vi "VCSV-Code-Program.vi"() -> ()   [LabVIEW 2018]
uses:
  <vilib>/sound2/lvsound2.llb/Sound Data Format.ctl
  <vilib>/sound2/lvsound2.llb/Sampling Mode.ctl
  <vilib>/userdefined/High Color/IMAQdx.ctl
  <vilib>/Analysis/3filter.llb/Filter Passband Type.ctl
  <vilib>/Analysis/2dsp.llb/Real FFT.vi
  <vilib>/Analysis/2dsp.llb/Inverse Real FFT.vi
  <vilib>/sound2/lvsound2.llb/Sound Input Read (DBL).vi
  <vilib>/Analysis/3filter.llb/Butterworth Filter (DBL).vi
  <vilib>/imath/engines/lvmath2/RunTimeEngine/BuiltInFunctions/length/NIMS_length(GV).vi
  <instcachedir>/0/NIMS_length(GV)_08A3D13377FD4E4B96F5795FBF3698FA.lvgen/NIMS_length(GV)_08A3D13377FD4E4B96F5795FBF3698FA_000.vi
  <vilib>/imath/engines/lvmath2/RunTimeEngine/CommandStatement/MC_CommandStatement_break.vi
  <vilib>/imath/engines/lvmath2/RunTimeEngine/IndexRead/NIMS V(S).vi
  <instcachedir>/0/NIMS V(S)_0488751826AF41519A22953C041130DC.lvgen/NIMS V(S)_0488751826AF41519A22953C041130DC_000.vi
  <vilib>/imathl/engines/lvmath/Functions/Error Handling/Create Error.vi
  <vilib>/imath/engines/lvmath2/RunTimeEngine/CommandStatement/NIMS_CommandStatement_MaskErr.vi
  <vilib>/imath/engines/lvmath2/RunTimeEngine/NodeEndStatement/NIMS_NodeEndStatement_Output.vi
  <instcachedir>/0/NIMS_NodeEndStatement_Output_53EC0D466D134D7ABD903AC30B43404B.lvgen/NIMS_NodeEndStatement_Output_53EC0D466D134D7ABD903AC30B43404B_010.vi
  <instcachedir>/0/NIMS_NodeEndStatement_Output_53EC0D466D134D7ABD903AC30B43404B.lvgen/NIMS_NodeEndStatement_Output_53EC0D466D134D7ABD903AC30B43404B_009.vi
  <vilib>/imath/engines/lvmath2/RunTimeEngine/ErrorHandling/NIMS_Finalize Error.vi
  <vilib>/Analysis/2dsp.llb/Zero Padder (DBL).vi
  <vilib>/imath/engines/lvmath2/RunTimeEngine/Managers/WorkSpace/UID Generator.vi
  <vilib>/imath/engines/lvmath2/RunTimeEngine/RunTimeType/NIMS_RunTimeType_From StrictType (excl LVString).vi
  <instcachedir>/0/NIMS_RunTimeType_From StrictType (excl LVString)_E7E34A65C99947108168652BAD14964D.lvgen/NIMS_RunTimeType_From StrictType (excl LVString)_E7E34A65C99947108168652BAD14964D_000.vi
  <vilib>/imath/engines/lvmath2/RunTimeEngine/LocalVariableDefStatement/MC_LocalVariableDefStatement_Display.vi
  <vilib>/imath/engines/lvmath2/RunTimeEngine/Managers/SymbolTable/Clear UID.vi
  <vilib>/Analysis/NI_AALBase.lvlib
  <vilib>/Analysis/NI_AALPro.lvlib
  <vilib>/imath/engines/lvmath2/RunTimeEngine/Managers/SymbolTable/NIMS_WorkSpace.lvlib
  <vilib>/vision/driver/NI_Vision_Acquisition_Software.lvlib
panel:
  in  "temp":dbl=25.0
  in  "stop":bool
  out "X":dbl
  out "Y":dbl
  out "Z":dbl
  out "theta":dbl
  out "phi":dbl
  out "c 2":i32
  in  "Hide/Show (Show)":bool=TRUE
  in  "Bring To Front? (N)":bool
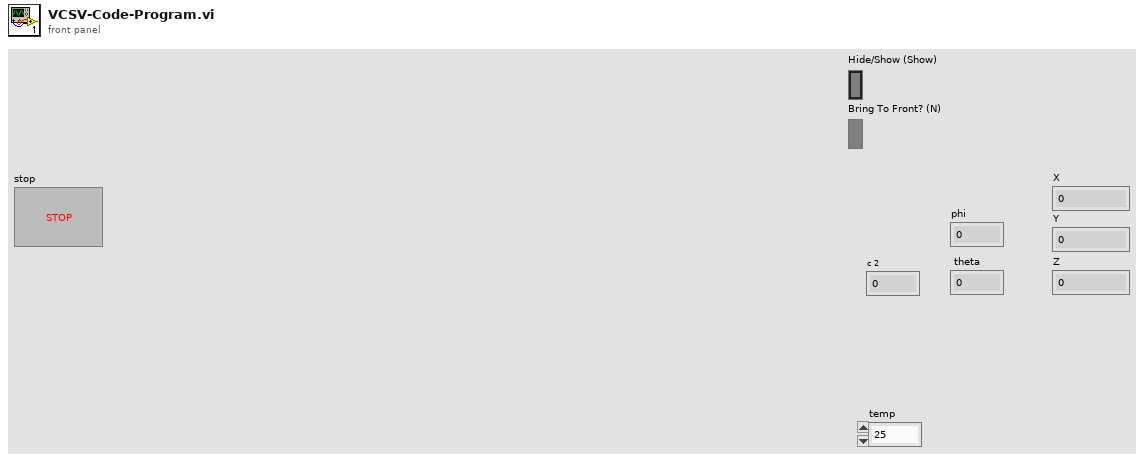
[diagram p1: front panel]
types:
  T1 = typedef "IMAQdx.ctl" = refnum<k21>
  T2 = typedef "Sampling Mode.ctl" = i32
  T3 = typedef "Sound Data Format.ctl" = cluster{"sample rate (S/s)":dbl, "number of channels":i32, "bits per sample":i32}
  T4 = typedef "Sound Input Task ID.ctl" = u32
  T5 = typedef "NI_AALBase.lvlib/Filter Passband Type.ctl" = enum32{"Lowpass", "Highpass", "Bandpass", "Bandstop"}
  T6 = typedef "IMAQ Image.ctl" = refnum<image>
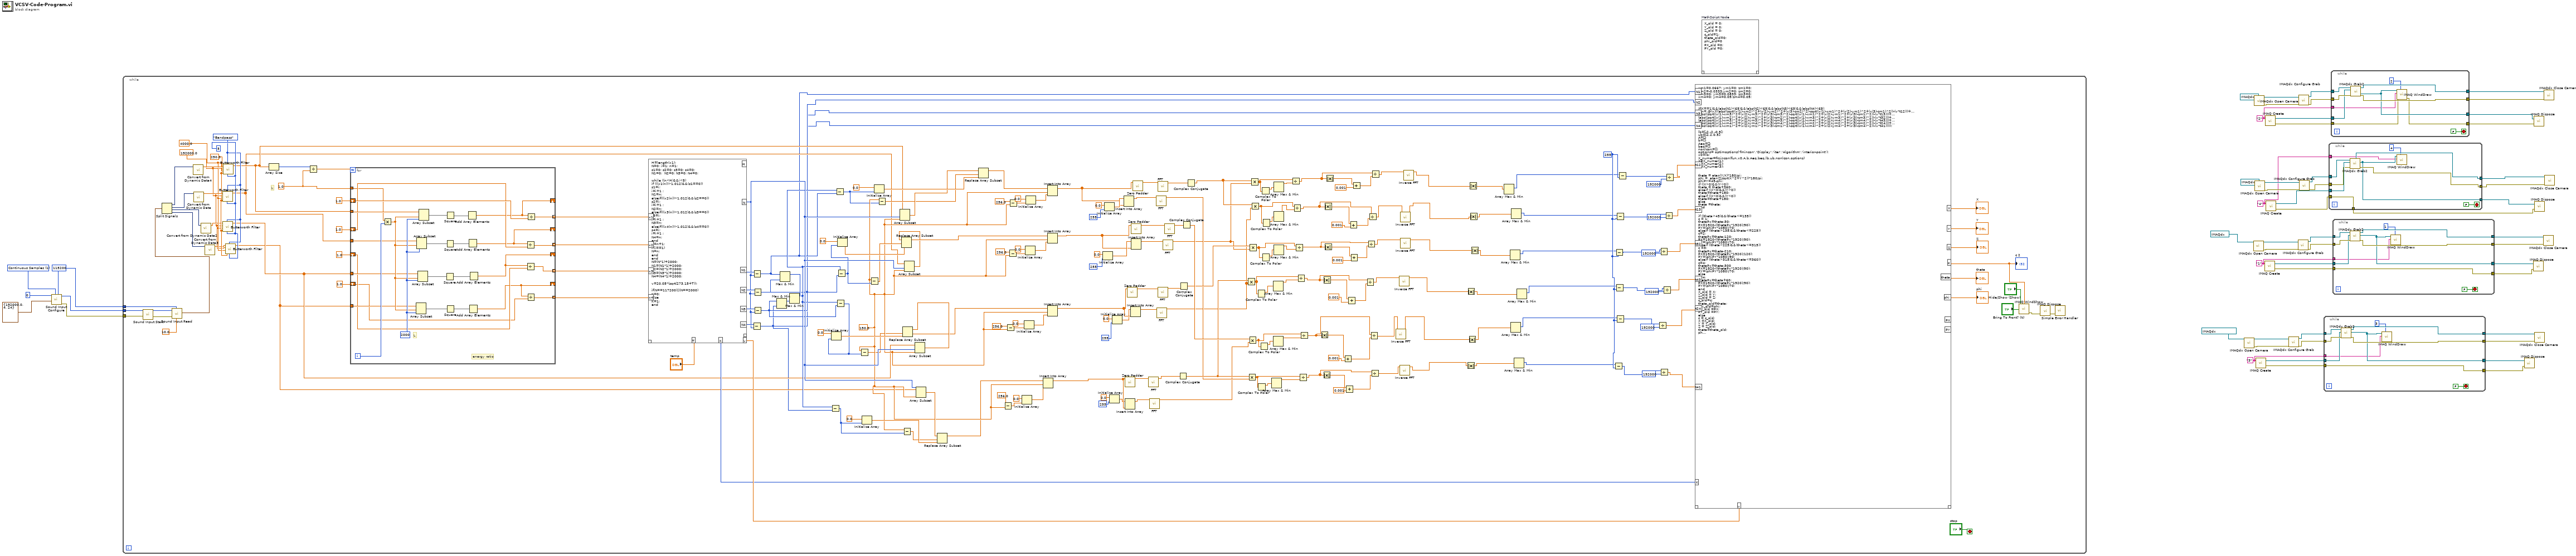
[diagram p0: block diagram]
diagram:
  w1 = "3" ("Image Name")
  w15 = "2" ("Image Name")
  w14 = "4" ("Image Name")
  w13 = "1" ("Image Name")
  w53 = T2 1 items=["Finite Samples", "Continuous Samples"] ("sample mode")
  w51 = 115200 ("number of samples/ch")
  n1 = call <vilib>:"Sound Input Configure.vi"("number of samples/ch"=w51, "sample mode"=w53, "sound format"=T3 {"sample rate (S/s)"=192000.0, "number of channels"=4, "bits per sample"=24}, "device ID"=u32 0) -> ("error out"=w50:errorcluster, "task ID"=w49:T4)  [unwired: 6 in]
  n2 = while {
    tunnel: w51 -> [w272]
    tunnel: w50 -> [w271]
    tunnel: w49 -> [w270]
    stop <- "stop" stop-if-true
    w65 = 1.0 ("x")
    w119 = 150.0
    w150 = 4000.0 ("high cutoff freq: fh")
    w151 = 250.0 ("low cutoff freq: fl")
    w152 = 5 ("order")
    w147 = 192000.0 ("sampling freq: fs")
    w146 = Filter_Passband_Type."Bandpass" ("filter type")
    w164 = 255
    # "k"
    n3 = call <vilib>:"Sound Input Start.vi"("error in (no error)"=w271, "task ID"=w270) -> ("error out"=w275:errorcluster, "task ID out"=w274:T4)  [unwired: 8 in]
    n4 = call-poly <vilib>:"Sound Input Read.vi"("timeout (sec)"=10.0, "number of samples/ch"=w272, "error in (no error)"=w275, "task ID"=w274) -> ("data"=w157:waveform(dbl)[])  [unwired: 5 in, 2 out]
    n5 = Split Signals(w157) -> (w277:dynamicdata, w156:dynamicdata, w155:dynamicdata, w158:dynamicdata)  [unwired: 4 in]
    n6 = call "Convert from Dynamic Data4"("Dynamic Data Type"=w277) -> ("Array"=w154:dbl[])  [unwired: 3 in]
    n7 = call "Convert from Dynamic Data"("Dynamic Data Type"=w156) -> ("Array"=w153:dbl[])  [unwired: 3 in]
    n8 = call "Convert from Dynamic Data2"("Dynamic Data Type"=w155) -> ("Array"=w149:dbl[])  [unwired: 3 in]
    n9 = call "Convert from Dynamic Data3"("Dynamic Data Type"=w158) -> ("Array"=w148:dbl[])  [unwired: 3 in]
    n10 = call-poly <vilib>:"Butterworth Filter.vi"("order"=w152, "filter type"=w146, "low cutoff freq: fl"=w151, "high cutoff freq: fh"=w150, "sampling freq: fs"=w147, "X"=w153) -> ("Filtered X"=w99:dbl[])  [unwired: 2 in, 1 out]
    n11 = call-poly <vilib>:"Butterworth Filter.vi"("order"=w152, "filter type"=w146, "low cutoff freq: fl"=w151, "high cutoff freq: fh"=w150, "sampling freq: fs"=w147, "X"=w149) -> ("Filtered X"=w98:dbl[])  [unwired: 2 in, 1 out]
    n12 = call-poly <vilib>:"Butterworth Filter.vi"("order"=w152, "filter type"=w146, "low cutoff freq: fl"=w151, "high cutoff freq: fh"=w150, "sampling freq: fs"=w147, "X"=w154) -> ("Filtered X"=w100:dbl[])  [unwired: 2 in, 1 out]
    n13 = call-poly <vilib>:"Butterworth Filter.vi"("order"=w152, "filter type"=w146, "low cutoff freq: fl"=w151, "high cutoff freq: fh"=w150, "sampling freq: fs"=w147, "X"=w148) -> ("Filtered X"=w97:dbl[])  [unwired: 2 in, 1 out]
    n14 = Array Size(array=w100) -> (size(s)=w66:i32)
    n15 = Divide(x=w66, y=w65) -> (x/y=w64:dbl)
    n16 = for {
      N: w64 -> [_]
      tunnel: w100 -> [w305]
      shift-right: [w285] -> _
      shift-left: 1.0 -> [w304]
      tunnel: [w303] -> w104 mode=indexing
      tunnel: w99 -> [w296]
      tunnel: w98 -> [w297]
      tunnel: w97 -> [w298]
      shift-right: [w283] -> _
      shift-left: 1.0 -> [w292]
      tunnel: [w291] -> w103 mode=indexing
      shift-right: [w281] -> _
      shift-left: 1.0 -> [w290]
      tunnel: [w289] -> w102 mode=indexing
      shift-right: [w279] -> _
      shift-left: 1.0 -> [w287]
      tunnel: [w288] -> w101 mode=indexing
      tunnel: w65 -> [w278]
      i -> [w301]
      w300 = 2000 ("length")
      # "energy ratio"
      # "L"
      n17 = Multiply(x=w278, y=w301) -> (x*y=w299:dbl)
      n18 = Array Subset "Array Subset"(array=w298, index=w299, length=w300) -> (w293:dbl[])
      n19 = Array Subset "Array Subset"(array=w296, index=w299, length=w300) -> (w295:dbl[])
      n20 = Array Subset "Array Subset"(array=w297, index=w299, length=w300) -> (w294:dbl[])
      n21 = Array Subset "Array Subset"(array=w305, index=w299, length=w300) -> (w302:dbl[])
      n22 = Square(x=w294) -> (x^2=w282:dbl[])
      n23 = Square(x=w295) -> (x^2=w284:dbl[])
      n24 = Square(x=w302) -> (x^2=w286:dbl[])
      n25 = Square(x=w293) -> (x^2=w280:dbl[])
      n26 = Add Array Elements(numeric array=w286) -> (sum=w285:dbl)
      n27 = Add Array Elements(numeric array=w284) -> (sum=w283:dbl)
      n28 = Add Array Elements(numeric array=w280) -> (sum=w279:dbl)
      n29 = Add Array Elements(numeric array=w282) -> (sum=w281:dbl)
      n30 = Divide(x=w283, y=w292) -> (x/y=w291:dbl)
      n31 = Divide(x=w281, y=w290) -> (x/y=w289:dbl)
      n32 = Divide(x=w279, y=w287) -> (x/y=w288:dbl)
      n33 = Divide(x=w285, y=w304) -> (x/y=w303:dbl)
    }
    n34 = mathscript code="H=length(x1);\nN=0; i=1; n=1;\ns1=0; s2=0; s3=0; s4=0;\nN1=0;  N2=0; N3=0; N4=0;\n\nwhile ((n<H)&&i<5)\nif (((x1(n))>1.012)&&(s1==0))\ns1=i;\ni=i+1 ;\nN1=n;\nelseif(((x2(n))>1.012)&&(s2==0))\ns2=i;\ni=i+1 ;\nN2=n;\nelseif(((x3(n))>1.012)&&(s3==0))\ns3=i;\ni=i+1 ;\nN3=n;\nelseif(((x4(n))>1.012)&&(s4==0))\ns4=i;\ni=i+1 ;\nN4=n;\nend\nn=n+1;\nif(i==1)\nN=n;\nend\nend\nN=(N*1)+2000;\nN1=(N1*1)+2000;\nN2=(N2*1)+2000;\nN3=(N3*1)+2000;\nN4=(N4*1)+2000;\n\nv=20.05*(sqrt(273.15+T));\n\nif(N==117200)||(N==2000)\nK=0;\nelse\nK=1;\nend"("x1"=w104, "x2"=w103, "x3"=w102, "x4"=w101, "T"="temp") -> ("N"=w128:i32, "v"=w145:cdb, "N1"=w132:i32, "N2"=w131:i32, "N3"=w130:i32, "N4"=w129:i32, "K"=w111:i32)  [unwired: 1 in, 2 out]
    n35 = Subtract(x=w129, y=w128) -> (x-y=w67:i32)
    n36 = Subtract(x=w132, y=w128) -> (x-y=w70:i32)
    n37 = Subtract(x=w131, y=w128) -> (x-y=w69:i32)
    n38 = Subtract(x=w130, y=w128) -> (x-y=w68:i32)
    n39 = Max & Min(x=w68, y=w67) -> (max(x,y)=w127:i32)  [unwired: 1 out]
    n40 = Max & Min(x=w70, y=w69) -> (max(x,y)=w126:i32)  [unwired: 1 out]
    n41 = Max & Min(x=w126, y=w127) -> (max(x,y)=w125:i32)  [unwired: 1 out]
    n42 = Subtract(x=w125, y=w67) -> (x-y=w124:i32)
    n43 = Subtract(x=w125, y=w70) -> (x-y=w118:i32)
    n44 = Subtract(x=w125, y=w68) -> (x-y=w122:i32)
    n45 = Initialize Array "Initialize Array"(0.0 ("element"), w122) -> (w137:dbl[])
    n46 = Subtract(x=w125, y=w69) -> (x-y=w121:i32)
    n47 = Initialize Array "Initialize Array"(0.0 ("element"), w121) -> (w139:dbl[])
    n48 = Subtract(x=w119, y=w122) -> (x-y=w116:dbl)
    n49 = Initialize Array "Initialize Array"(0.0 ("element"), w124) -> (w133:dbl[])
    n50 = Subtract(x=w119, y=w121) -> (x-y=w120:dbl)
    n51 = Initialize Array "Initialize Array"(0.0 ("element"), w118) -> (w142:dbl[])
    n52 = Subtract(x=w119, y=w118) -> (x-y=w117:dbl)
    n53 = Array Subset "Array Subset"(array=w100, index=w128, length=w119) -> (w141:dbl[])
    n54 = Subtract(x=w119, y=w124) -> (x-y=w123:dbl)
    n55 = Array Subset "Array Subset"(array=w99, index=w128, length=w119) -> (w105:dbl[])
    n56 = Replace Array Subset(array=w105, new element=w139, index=w120) -> (w113:dbl[])
    n57 = Array Subset "Array Subset"(array=w98, index=w128, length=w119) -> (w134:dbl[])
    n58 = Replace Array Subset(array=w134, new element=w137, index=w116) -> (w114:dbl[])
    n59 = Array Subset "Array Subset"(array=w97, index=w128, length=w119) -> (w135:dbl[])
    n60 = Replace Array Subset "Replace Array Subset"(array=w135, new element=w133, index=w123) -> (w115:dbl[])
    n61 = Replace Array Subset "Replace Array Subset"(array=w141, new element=w142, index=w117) -> (w112:dbl[])
    n62 = Subtract(x=256.0, y=w119) -> (x-y=w267:dbl)
    n63 = Subtract(x=256.0, y=w119) -> (x-y=w268:dbl)
    n64 = Subtract(x=256.0, y=w119) -> (x-y=w266:dbl)
    n65 = Subtract(x=256.0, y=w119) -> (x-y=w269:dbl)
    n66 = Initialize Array(0.0 ("element"), w267) -> (w254:dbl[])
    n67 = Initialize Array(0.0 ("element"), w268) -> (w257:dbl[])
    n68 = Initialize Array(0.0 ("element"), w266) -> (w256:dbl[])
    n69 = Initialize Array(0.0 ("element"), w269) -> (w255:dbl[])
    n70 = Insert Into Array "Insert Into Array"(array=w115, index=w119, new element=w254) -> (w234:dbl[])
    n71 = Insert Into Array(array=w113, index=w119, new element=w256) -> (w238:dbl[])
    n72 = Insert Into Array(array=w112, index=w119, new element=w255) -> (w252:dbl[])
    n73 = Insert Into Array(array=w114, index=w119, new element=w257) -> (w236:dbl[])
    n74 = Initialize Array(0.0 ("element"), 255 ("dimension size")) -> (w239:dbl[])
    n75 = Initialize Array(0.0 ("element"), 255 ("dimension size")) -> (w253:dbl[])
    n76 = Initialize Array(0.0 ("element"), 255 ("dimension size")) -> (w233:dbl[])
    n77 = Initialize Array(0.0 ("element"), 255 ("dimension size")) -> (w235:dbl[])
    n78 = Insert Into Array(array=w253, new element=w252) -> (w242:dbl[])  [unwired: 1 in]
    n79 = call-poly <vilib>:"Zero Padder.vi"("Input Array"=w234) -> ("Zero Padded Array"=w230:dbl[])  [unwired: 10 in]
    n80 = Insert Into Array(array=w233, new element=w234) -> (w232:dbl[])  [unwired: 1 in]
    n81 = call-poly <vilib>:"Zero Padder.vi"("Input Array"=w236) -> ("Zero Padded Array"=w237:dbl[])  [unwired: 10 in]
    n82 = Insert Into Array(array=w235, new element=w236) -> (w231:dbl[])  [unwired: 1 in]
    n83 = call-poly <vilib>:"Zero Padder.vi"("Input Array"=w238) -> ("Zero Padded Array"=w241:dbl[])  [unwired: 10 in]
    n84 = Insert Into Array(array=w239, new element=w238) -> (w240:dbl[])  [unwired: 1 in]
    n85 = call-poly <vilib>:"Zero Padder.vi"("Input Array"=w252) -> ("Zero Padded Array"=w243:dbl[])  [unwired: 10 in]
    n86 = call-poly <vilib>:"FFT.vi"("X"=w230) -> ("FFT {X}"=w228:cdb[])  [unwired: 9 in, 1 out]
    n87 = call-poly <vilib>:"FFT.vi"("X"=w232) -> ("FFT {X}"=w213:cdb[])  [unwired: 9 in, 1 out]
    n88 = call-poly <vilib>:"FFT.vi"("X"=w242) -> ("FFT {X}"=w215:cdb[])  [unwired: 9 in, 1 out]
    n89 = call-poly <vilib>:"FFT.vi"("X"=w231) -> ("FFT {X}"=w214:cdb[])  [unwired: 9 in, 1 out]
    n90 = call-poly <vilib>:"FFT.vi"("X"=w243) -> ("FFT {X}"=w229:cdb[])  [unwired: 9 in, 1 out]
    n91 = call-poly <vilib>:"FFT.vi"("X"=w237) -> ("FFT {X}"=w227:cdb[])  [unwired: 9 in, 1 out]
    n92 = call-poly <vilib>:"FFT.vi"("X"=w240) -> ("FFT {X}"=w110:cdb[])  [unwired: 9 in, 1 out]
    n93 = call-poly <vilib>:"FFT.vi"("X"=w241) -> ("FFT {X}"=w226:cdb[])  [unwired: 9 in, 1 out]
    n94 = Complex Conjugate(1:w228) -> (0:w217:cdb[])
    n95 = Complex Conjugate(1:w227) -> (0:w218:cdb[])
    n96 = Complex Conjugate(1:w226) -> (0:w219:cdb[])
    n97 = Complex Conjugate(1:w229) -> (0:w216:cdb[])
    n98 = Multiply(x=w217, y=w214) -> (x*y=w207:cdb[])
    n99 = Multiply(x=w217, y=w215) -> (x*y=w212:cdb[])
    n100 = Multiply(x=w219, y=w213) -> (x*y=w209:cdb[])
    n101 = Multiply(x=w218, y=w110) -> (x*y=w205:cdb[])
    n102 = Multiply(x=w216, y=w110) -> (x*y=w201:cdb[])
    n103 = Multiply(x=w216, y=w214) -> (x*y=w203:cdb[])
    n104 = Complex To Polar(r * e^(i*theta)=w207) -> (r=w223:dbl[])  [unwired: 1 out]
    n105 = Complex To Polar(r * e^(i*theta)=w212) -> (r=w225:dbl[])  [unwired: 1 out]
    n106 = Complex To Polar(r * e^(i*theta)=w209) -> (r=w224:dbl[])  [unwired: 1 out]
    n107 = Complex To Polar(r * e^(i*theta)=w201) -> (r=w220:dbl[])  [unwired: 1 out]
    n108 = Complex To Polar(r * e^(i*theta)=w205) -> (r=w222:dbl[])  [unwired: 1 out]
    n109 = Complex To Polar(r * e^(i*theta)=w203) -> (r=w221:dbl[])  [unwired: 1 out]
    n110 = Array Max & Min(array=w225) -> (max value=w211:dbl)  [unwired: 3 out]
    n111 = Array Max & Min(array=w223) -> (max value=w208:dbl)  [unwired: 3 out]
    n112 = Array Max & Min(array=w224) -> (max value=w210:dbl)  [unwired: 3 out]
    n113 = Array Max & Min(array=w220) -> (max value=w202:dbl)  [unwired: 3 out]
    n114 = Array Max & Min(array=w221) -> (max value=w204:dbl)  [unwired: 3 out]
    n115 = Array Max & Min(array=w222) -> (max value=w206:dbl)  [unwired: 3 out]
    n116 = Divide(x=w201, y=w202) -> (x/y=w199:cdb[])
    n117 = Divide(x=w203, y=w204) -> (x/y=w194:cdb[])
    n118 = Divide(x=w205, y=w206) -> (x/y=w195:cdb[])
    n119 = Divide(x=w207, y=w208) -> (x/y=w196:cdb[])
    n120 = Divide(x=w212, y=w211) -> (x/y=w198:cdb[])
    n121 = Divide(x=w209, y=w210) -> (x/y=w197:cdb[])
    n122 = Absolute Value(x=w197) -> (abs(x)=w187:dbl[])
    n123 = Absolute Value(x=w198) -> (abs(x)=w185:dbl[])
    n124 = Absolute Value(x=w196) -> (abs(x)=w189:dbl[])
    n125 = Absolute Value(x=w194) -> (abs(x)=w193:dbl[])
    n126 = Absolute Value(x=w195) -> (abs(x)=w191:dbl[])
    n127 = Absolute Value(x=w199) -> (abs(x)=w200:dbl[])
    n128 = Add(x=w187, y=0.001) -> (x+y=w186:dbl[])
    n129 = Add(x=w185, y=0.001) -> (x+y=w184:dbl[])
    n130 = Add(x=w189, y=0.001) -> (x+y=w188:dbl[])
    n131 = Add(x=w193, y=0.001) -> (x+y=w192:dbl[])
    n132 = Add(x=w191, y=0.001) -> (x+y=w190:dbl[])
    n133 = Add(x=w200, y=0.001) -> (x+y=w177:dbl[])
    n134 = Divide(x=w196, y=w188) -> (x/y=w174:cdb[])
    n135 = Divide(x=w195, y=w190) -> (x/y=w173:cdb[])
    n136 = Divide(x=w194, y=w192) -> (x/y=w172:cdb[])
    n137 = Divide(x=w197, y=w186) -> (x/y=w175:cdb[])
    n138 = Divide(x=w198, y=w184) -> (x/y=w176:cdb[])
    n139 = Divide(x=w199, y=w177) -> (x/y=w171:cdb[])
    n140 = call-poly <vilib>:"Inverse FFT.vi"("FFT {X}"=w175) -> ("X"=w166:dbl[])  [unwired: 9 in, 1 out]
    n141 = call-poly <vilib>:"Inverse FFT.vi"("FFT {X}"=w174) -> ("X"=w167:dbl[])  [unwired: 9 in, 1 out]
    n142 = call-poly <vilib>:"Inverse FFT.vi"("FFT {X}"=w176) -> ("X"=w165:dbl[])  [unwired: 9 in, 1 out]
    n143 = call-poly <vilib>:"Inverse FFT.vi"("FFT {X}"=w172) -> ("X"=w169:dbl[])  [unwired: 9 in, 1 out]
    n144 = call-poly <vilib>:"Inverse FFT.vi"("FFT {X}"=w173) -> ("X"=w168:dbl[])  [unwired: 9 in, 1 out]
    n145 = call-poly <vilib>:"Inverse FFT.vi"("FFT {X}"=w171) -> ("X"=w170:dbl[])  [unwired: 9 in, 1 out]
    n146 = Absolute Value(x=w165) -> (abs(x)=w86:dbl[])
    n147 = Absolute Value(x=w167) -> (abs(x)=w90:dbl[])
    n148 = Absolute Value(x=w166) -> (abs(x)=w88:dbl[])
    n149 = Absolute Value(x=w170) -> (abs(x)=w96:dbl[])
    n150 = Absolute Value(x=w169) -> (abs(x)=w94:dbl[])
    n151 = Absolute Value(x=w168) -> (abs(x)=w92:dbl[])
    n152 = Array Max & Min(array=w96) -> (max index (indices)=w95:i32)  [unwired: 3 out]
    n153 = Array Max & Min(array=w92) -> (max index (indices)=w91:i32)  [unwired: 3 out]
    n154 = Array Max & Min(array=w88) -> (max index (indices)=w87:i32)  [unwired: 3 out]
    n155 = Array Max & Min(array=w94) -> (max index (indices)=w93:i32)  [unwired: 3 out]
    n156 = Array Max & Min(array=w86) -> (max index (indices)=w85:i32)  [unwired: 3 out]
    n157 = Array Max & Min(array=w90) -> (max index (indices)=w89:i32)  [unwired: 3 out]
    n158 = Subtract(x=w85, y=w164) -> (x-y=w72:i32)
    n159 = Subtract(x=w91, y=w164) -> (x-y=w79:i32)
    n160 = Subtract(x=w89, y=w164) -> (x-y=w77:i32)
    n161 = Subtract(x=w93, y=w164) -> (x-y=w82:i32)
    n162 = Subtract(x=w87, y=w164) -> (x-y=w75:i32)
    n163 = Subtract(x=w95, y=w164) -> (x-y=w84:i32)
    n164 = Divide(x=w75, y=192000) -> (x/y=w74:dbl)
    n165 = Divide(x=w79, y=192000) -> (x/y=w60:dbl)
    n166 = Divide(x=w72, y=192000) -> (x/y=w62:dbl)
    n167 = Divide(x=w77, y=192000) -> (x/y=w63:dbl)
    n168 = Divide(x=w82, y=192000) -> (x/y=w81:dbl)
    n169 = Divide(x=w84, y=192000) -> (x/y=w61:dbl)
    n170 = script code="xm1=0.0667; ym1=0; zm1=0;\nxm2=-0.0333;ym2=0; zm2=0;\nxm3=0; ym3=0.0833; zm3=0;\nxm4=0; ym4=0.05;zm4=0.05;\n\n\n\nif(K==1)&&(abs(N1)<65)&&(abs(N2)<65)&&(abs(N3)<65)&&(abs(N4)<65)\nfun= @(x)(((abs((sqrt((x(1)-xm2)^2+(x(2)-ym2)^2+(x(3)-zm2)^2)-sqrt((x(1)-xm1)^2+(x(2)-ym1)^2+(x(3)-zm1)^2))-(v*t12)))+...\n(abs((sqrt((x(1)-xm3)^2+(x(2)-ym3)^2+(x(3)-zm3)^2)-sqrt((x(1)-xm1)^2+(x(2)-ym1)^2+(x(3)-zm1)^2))-(v*t13)))+...\n(abs((sqrt((x(1)-xm2)^2+(x(2)-ym2)^2+(x(3)-zm2)^2)-sqrt((x(1)-xm3)^2+(x(2)-ym3)^2+(x(3)-zm3)^2))-(v*t32)))+...\n(abs((sqrt((x(1)-xm3)^2+(x(2)-ym3)^2+(x(3)-zm3)^2)-sqrt((x(1)-xm4)^2+(x(2)-ym4)^2+(x(3)-zm4)^2))-(v*t43)))+...\n(abs((sqrt((x(1)-xm4)^2+(x(2)-ym4)^2+(x(3)-zm4)^2)-sqrt((x(1)-xm2)^2+(x(2)-ym2)^2+(x(3)-zm2)^2))-(v*t24)))+...\n(abs((sqrt((x(1)-xm1)^2+(x(2)-ym1)^2+(x(3)-zm1)^2)-sqrt((x(1)-xm4)^2+(x(2)-ym4)^2+(x(3)-zm4)^2))-(v*t41)))));\n\nlb=[-2,-2,-0.5];\nub=[2,2,0.5];\nA=[];\nb=[];\nAeq=[];\nbeq=[];\nnonlcon=[];\noptions= optimoptions('fmincon','Display','iter','Algorithm','interior-point');\nx0=lb;\nX_numer=fmincon(fun,x0,A,b,Aeq,beq,lb,ub,nonlcon,options)\nX=X_numer(1);\nY=X_numer(2);\nZ=X_numer(3);\n\n\ntheta = atan(Y/X)*180/pi;\nphi =  atan(Z/sqrt(X^2+Y^2))*180/pi;\nphiPY=45-phi;\nif ((X>0)&&(Y<0))\ntheta = theta+360;\nelseif ((X<0)&&(Y>0))\ntheta=theta+180;\nelseif ((X<0)&&(Y<0))\ntheta=theta+180;\nelse \ntheta =theta;\nend\n\n\nif ((theta>45)&&(theta<=135))\nc = 1;\nthetaPx=theta-30;\nPX=1920-((thetaPx*1920)/90);\nPY=(phiPY*1080)/70;\nelseif ((theta>135)&&(theta<=225))\nc=2;\nthetaPx=theta-120;\nPX=1920-((thetaPx*1920)/90);\nPY=(phiPY*1080)/70;\nelseif ((theta>225)&&(theta<=315))\nc =3;\nthetaPx=theta-210;\nPX=1920-((thetaPx*1920)/120);\nPY=(phiPY*1080)/90;\nelseif ((theta>315)&&(theta<=360))\nc=4;\nthetaPx=theta-300\nPX=1920-((thetaPx*1920)/90);\nPY=(phiPY*1080)/70;\nelse\nc=4;\nthetaPx=theta+60;\nPX=1920-((thetaPx*1920)/90);\nPY=(phiPY*1080)/70;\nend\nX_old = X;\nY_old = Y;\nZ_old = Z;\nc_old=c;\ntheta_old=theta;\nphi_old=phi;\nPX_old =PX;\nPY_old =PY;\nelse\nc = c_old;\nX =X_old;\nY = Y_old;\nZ = Z_old;\ntheta=theta_old;\nphi=phi_old;\nPX =PX_old;\nPY =PY_old;\nend"("v"=w145, "t12"=w61, "t13"=w81, "t32"=w60, "t43"=w63, "t24"=w74, "t41"=w62, "K"=w111, "N1"=w70, "N2"=w69, "N3"=w68, "N4"=w67) -> ("X"=→"X":dbl, "Y"=→"Y":dbl, "Z"=→"Z":dbl, "c"=w55:dbl, "theta"=→"theta":dbl, "phi"=→"phi":dbl)  [unwired: 1 in, 3 out]
    "c 2" <- w55
    n171 = call "IMAQ WindShow"("Bring To Front? (N)"="Bring To Front? (N)", "Hide/Show (Show)"="Hide/Show (Show)", "Window Number (0...15)"=w55) -> ("error out"=w59:errorcluster)  [unwired: 3 in, 2 out]
    n172 = call "IMAQ Dispose"("error in (no error)"=w59) -> ("error out"=w58:errorcluster)  [unwired: 5 in]
    n173 = call <vilib>:"Simple Error Handler.vi"("error in (no error)"=w58) -> ()  [unwired: 4 in, 5 out]
  }
  n174 = mathscript code="X_old = 0;\nY_old = 0;\nZ_old = 0;\nc_old=1;\ntheta_old=0;\nphi_old=0\nPX_old =0;\nPY_old =0;"() -> ()  [unwired: 1 in, 1 out]
  n175 = call <vilib>:"IMAQdx Open Camera.vi"("Session In"=T1 "cam7") -> ("error out"=w12:errorcluster, "Session Out"=w11:T1)  [unwired: 9 in]
  n176 = call <vilib>:"IMAQdx Open Camera.vi"("Session In"=T1 "cam5") -> ("error out"=w38:errorcluster, "Session Out"=w37:T1)  [unwired: 9 in]
  n177 = call <vilib>:"IMAQdx Open Camera.vi"("Session In"=T1 "cam6") -> ("error out"=w48:errorcluster, "Session Out"=w47:T1)  [unwired: 9 in]
  n178 = call <vilib>:"IMAQdx Open Camera.vi"("Session In"=T1 "cam8") -> ("error out"=w41:errorcluster, "Session Out"=w40:T1)  [unwired: 9 in]
  n179 = call "IMAQ Create"("Image Name"=w1) -> ("New Image"=w2:T6, "error out"=w4:errorcluster)  [unwired: 4 in]
  n180 = call "IMAQ Create"("Image Name"=w13) -> ("New Image"=w22:T6, "error out"=w24:errorcluster)  [unwired: 4 in]
  n181 = call "IMAQ Create"("Image Name"=w15) -> ("New Image"=w42:T6, "error out"=w17:errorcluster)  [unwired: 4 in]
  n182 = call "IMAQ Create"("Image Name"=w14) -> ("New Image"=w39:T6, "error out"=w20:errorcluster)  [unwired: 4 in]
  n183 = call <vilib>:"IMAQdx Configure Grab.vi"("error in"=w12, "Session In"=w11) -> ("error out"=w9:errorcluster, "Session Out"=w10:T1)  [unwired: 8 in]
  n184 = call <vilib>:"IMAQdx Configure Grab.vi"("error in"=w38, "Session In"=w37) -> ("error out"=w35:errorcluster, "Session Out"=w36:T1)  [unwired: 8 in]
  n185 = call <vilib>:"IMAQdx Configure Grab.vi"("error in"=w48, "Session In"=w47) -> ("error out"=w45:errorcluster, "Session Out"=w46:T1)  [unwired: 8 in]
  n186 = call <vilib>:"IMAQdx Configure Grab.vi"("error in"=w41, "Session In"=w40) -> ("error out"=w26:errorcluster, "Session Out"=w29:T1)  [unwired: 8 in]
  n187 = while {
    tunnel: w10 -> [w879]
    tunnel: [w877] -> w8
    tunnel: w9 -> [w878]
    tunnel: [w876] -> w7
    tunnel: [w875] -> w5
    tunnel: w4 -> [w875]
    tunnel: [w873] -> w3
    tunnel: w2 -> [w874]
    tunnel: w1 -> [w872]
    stop <- FALSE stop-if-true
    n188 = call <vilib>:"IMAQdx Grab2.vi"("error in"=w878, "Image In"=w874, "Session In"=w879) -> ("error out"=w876:errorcluster, "Image Out"=w873:T6, "Session Out"=w877:T1)  [unwired: 5 in, 1 out]
    n189 = call "IMAQ WindDraw"("Window Number (0...15)"=3, "Title"=w872, "Image"=w873) -> ()  [unwired: 7 in, 2 out]
  }
  n190 = while {
    tunnel: w39 -> [w889]
    tunnel: w29 -> [w887]
    tunnel: [w886] -> w28
    tunnel: [w885] -> w27
    tunnel: w26 -> [w884]
    tunnel: [w882] -> w21
    tunnel: w20 -> [w883]
    tunnel: [w883] -> w19
    tunnel: w14 -> [w881]
    stop <- FALSE stop-if-true
    n191 = call <vilib>:"IMAQdx Grab2.vi"("error in"=w884, "Image In"=w889, "Session In"=w887) -> ("error out"=w885:errorcluster, "Image Out"=w882:T6, "Session Out"=w886:T1)  [unwired: 5 in, 1 out]
    n192 = call "IMAQ WindDraw"("Window Number (0...15)"=4, "Title"=w881, "Image"=w882) -> ()  [unwired: 7 in, 2 out]
  }
  n193 = while {
    tunnel: w42 -> [w896]
    tunnel: w46 -> [w900]
    tunnel: [w898] -> w44
    tunnel: w45 -> [w899]
    tunnel: [w897] -> w43
    tunnel: [w894] -> w18
    tunnel: w17 -> [w891]
    tunnel: [w890] -> w16
    tunnel: w15 -> [w892]
    stop <- FALSE stop-if-true
    n194 = call <vilib>:"IMAQdx Grab2.vi"("error in"=w899, "Image In"=w896, "Session In"=w900) -> ("error out"=w897:errorcluster, "Image Out"=w894:T6, "Session Out"=w898:T1)  [unwired: 5 in, 1 out]
    n195 = call "IMAQ WindDraw"("Window Number (0...15)"=2, "error in (no error)"=w891, "Title"=w892, "Image"=w894) -> ("error out"=w890:errorcluster)  [unwired: 6 in, 1 out]
  }
  n196 = while {
    tunnel: w36 -> [w910]
    tunnel: [w908] -> w34
    tunnel: w35 -> [w909]
    tunnel: [w907] -> w33
    tunnel: [w906] -> w25
    tunnel: w24 -> [w906]
    tunnel: [w904] -> w23
    tunnel: w22 -> [w905]
    tunnel: w13 -> [w903]
    stop <- FALSE stop-if-true
    n197 = call <vilib>:"IMAQdx Grab2.vi"("error in"=w909, "Image In"=w905, "Session In"=w910) -> ("error out"=w907:errorcluster, "Image Out"=w904:T6, "Session Out"=w908:T1)  [unwired: 5 in, 1 out]
    n198 = call "IMAQ WindDraw"("Window Number (0...15)"=1, "Title"=w903, "Image"=w904) -> ()  [unwired: 7 in, 2 out]
  }
  n199 = call "IMAQ Dispose"("Image"=w3, "error in (no error)"=w5) -> ()  [unwired: 4 in, 1 out]
  n200 = call "IMAQ Dispose"("Image"=w23, "error in (no error)"=w25) -> ()  [unwired: 4 in, 1 out]
  n201 = call "IMAQ Dispose"("Image"=w18, "error in (no error)"=w16) -> ()  [unwired: 4 in, 1 out]
  n202 = call <vilib>:"IMAQdx Close Camera.vi"("error in"=w7, "Session In"=w8) -> ()  [unwired: 9 in, 1 out]
  n203 = call "IMAQ Dispose"("Image"=w21, "error in (no error)"=w19) -> ()  [unwired: 4 in, 1 out]
  n204 = call <vilib>:"IMAQdx Close Camera.vi"("error in"=w33, "Session In"=w34) -> ()  [unwired: 9 in, 1 out]
  n205 = call <vilib>:"IMAQdx Close Camera.vi"("error in"=w43, "Session In"=w44) -> ()  [unwired: 9 in, 1 out]
  n206 = call <vilib>:"IMAQdx Close Camera.vi"("error in"=w27, "Session In"=w28) -> ()  [unwired: 9 in, 1 out]
